vi "dfd_Pi Complementary Lowpass to Highpass.vi"(1 "Lowpass":dbl[](array[numeric])) -> (0 "Highpass":dbl[](array[numeric]))   [LabVIEW 2017, in "NI_DigFilterLicensed.lvlib"]
uses:
  <vilib>/addons/Digital Filter Design/NI_DigFilterLicensed.lvlib
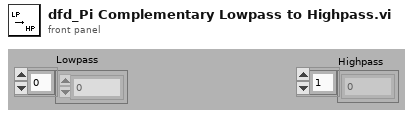
[diagram p1: front panel]
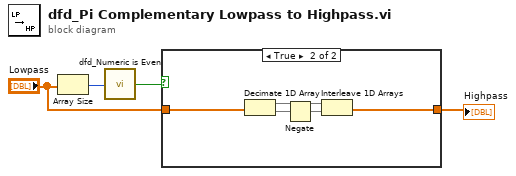
[diagram p0: block diagram]
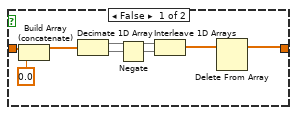
[diagram p2: hidden frame]
diagram:
  n1 = Array Size(array="Lowpass") -> (size(s)=w4:i32)
  n2 = call <vilib>:"dfd_Numeric is Even.vi"("N"=w4) -> ("even ?"=w3:bool)
  n3 = case shown="True" w3 {
    tunnel: [w5 w13] -> w1
    tunnel: "Lowpass" -> [w11 w14]
    frame False {
      n4 = Build Array (concatenate)(w11, 0.0) -> (w7:dbl[])
      n5 = Decimate 1D Array(w7) -> (w9:dbl[], w10:dbl[])
      n6 = Negate(x=w10) -> (-x=w8:dbl[])
      n7 = Interleave 1D Arrays(w9, w8) -> (w6:dbl[])
      n8 = Delete From Array(array=w6) -> (array with subset deleted=w5:dbl[])  [unwired: 2 in, 1 out]
    }
    frame True {
      n9 = Decimate 1D Array(w14) -> (w16:dbl[], w15:dbl[])
      n10 = Negate(x=w15) -> (-x=w17:dbl[])
      n11 = Interleave 1D Arrays(w16, w17) -> (w13:dbl[])
    }
  }
  "Highpass" <- w1
